vi "Triggered Tasks-Stop.vi"(8 "error in (no error)":errorcluster, 11 "Logging queue element":T1={"Imaging Protocol"=enum."Live Imaging", "Number of Trials"=0, "Frame Size"=512, "# Averaged frames"=0, "Dwell time (us)"=0.0, "Index of Z-plane"=0, "Timelapse?"=FALSE, "Logging process is active"=FALSE, "Speed logging enabled"=FALSE, "tdms file ref"=refnum, "path"=path "", "Trial Number"=0, "Expected # points acquired"=FALSE, "Manually stopped"=FALSE, "Last trial"=FALSE, "Ch0 data"=[], "Ch1 data"=[], "Ref Data"=[], "Ref Frame Time"=[], "Image Time"=[], "Continuous Time"=[], "Ref X Length"=0, "Ref Y Length"=0, "# Ref Averaged frames"=0, "Ref Dwell time (us)"=0.0, "Points acquired"={"Ch0 last trial"=0, "Ch1 last trial"=0, "All trials"=0}, "HW Timings File"=refnum} {"Ref Dwell time (us)" format="%#.6g"; "Frame Size" items=["100X100"=100, "128X128"=128, "200X200"=200, "256X256"=256, "512X512"=512, "1024x1024"=1024, "2048x2048"=2048]; "Dwell time (us)" format="%#.6g"}) -> (0 "error out":errorcluster)   [LabVIEW 2020]
uses:
  Typedefs/Logging queue element.ctl
  Typedefs/Imaging Protocols enum.ctl
  Typedefs/Frame Size.ctl
  Typedefs/Acquired points count.ctl
  Typedefs/Read Write Enum.ctl
  Typedefs/fgv_actions.ctl
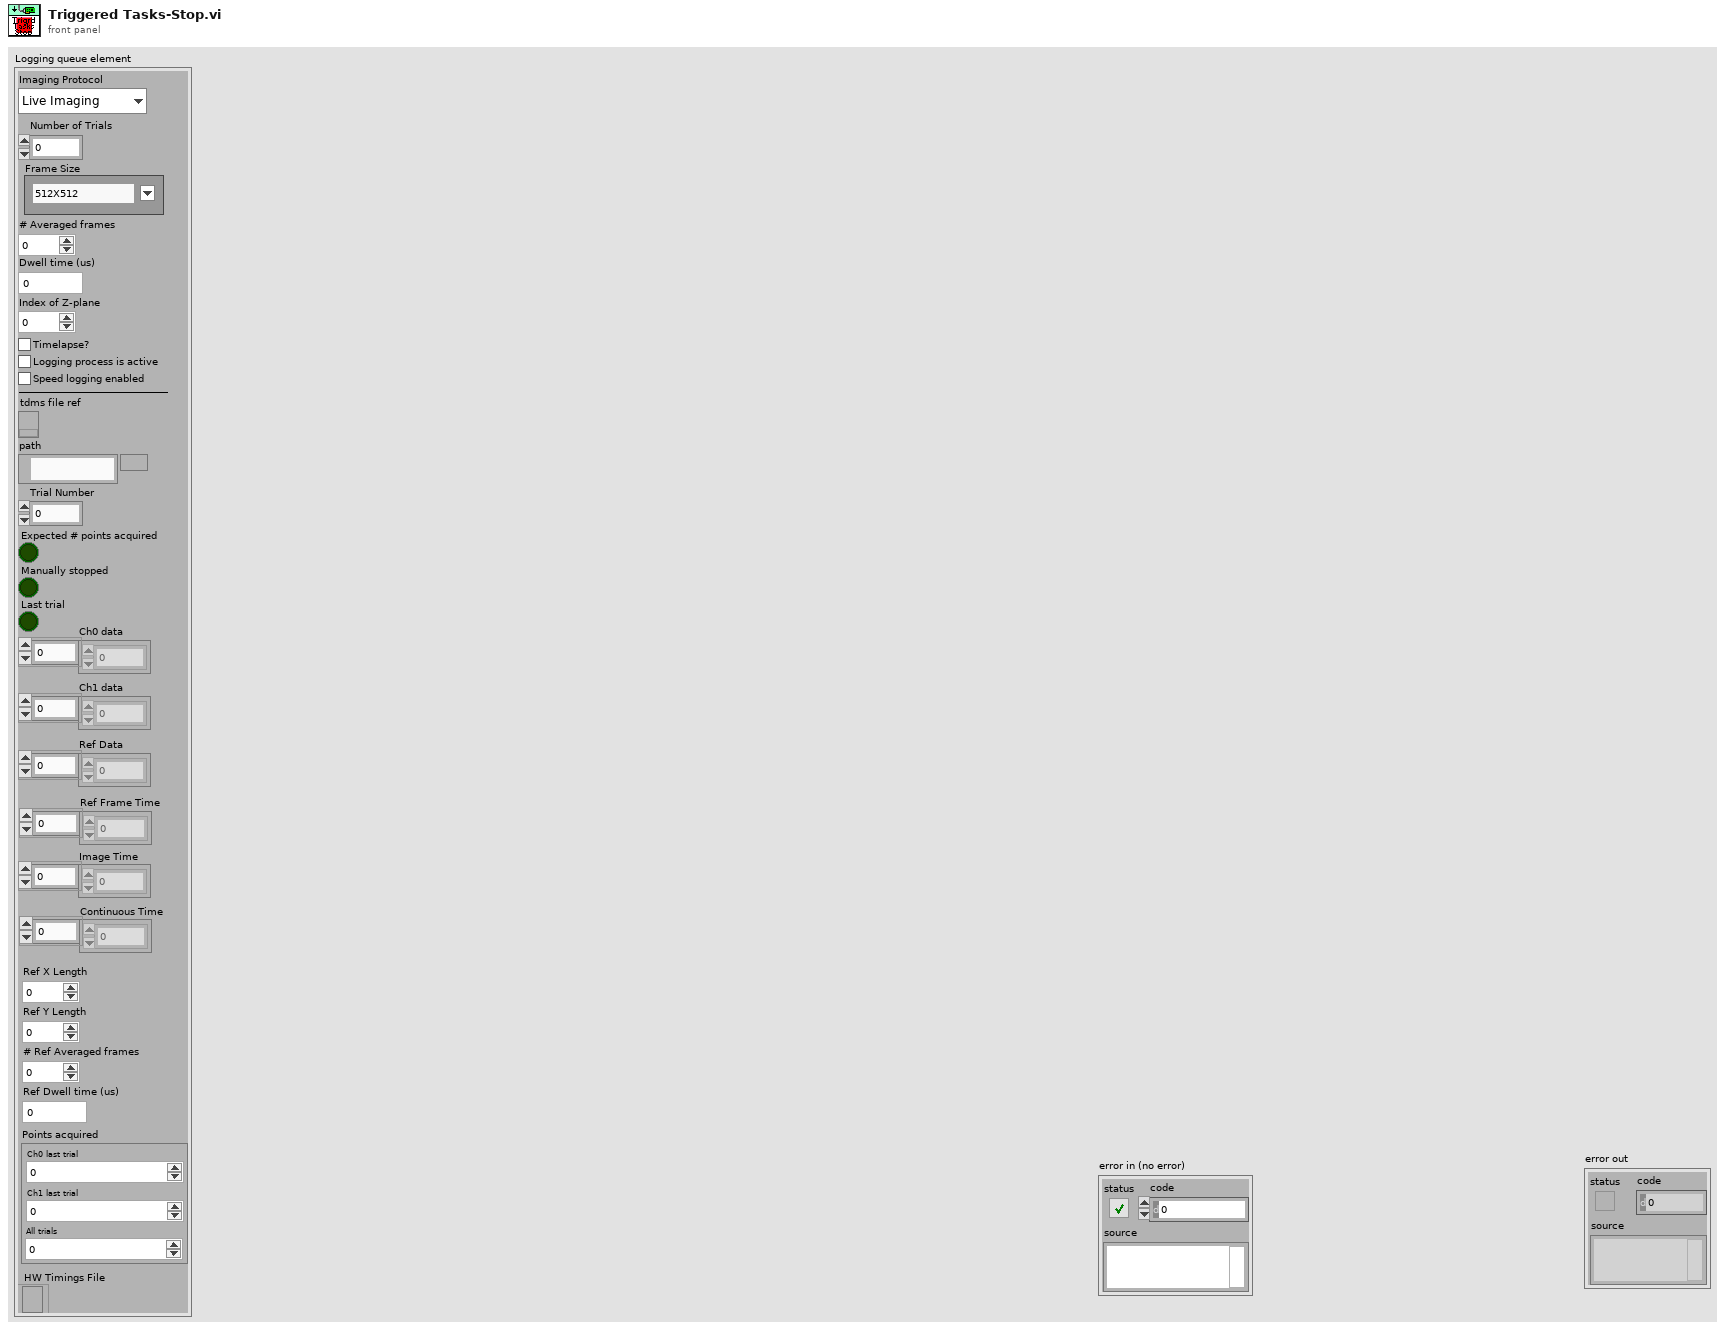
[diagram p1: front panel]
types:
  T1 = typedef "Logging queue element.ctl" = cluster{"Imaging Protocol":T2, "Number of Trials":u16, "Frame Size":T3, "# Averaged frames":u16, "Dwell time (us)":dbl, "Index of Z-plane":i32, "Timelapse?":bool, "Logging process is active":bool, "Speed logging enabled":bool, "tdms file ref":refnum<k34>, "path":path, "Trial Number":i32, "Expected # points acquired":bool, "Manually stopped":bool, "Last trial":bool, "Ch0 data":u32[], "Ch1 data":u32[], "Ref Data":u32[], "Ref Frame Time":u64[], "Image Time":u64[], "Continuous Time":u64[], "Ref X Length":u16, "Ref Y Length":u16, "# Ref Averaged frames":u16, "Ref Dwell time (us)":dbl, "Points acquired":T4, "HW Timings File":refnum<file>}
  T2 = typedef "Imaging Protocols enum.ctl" = enum16{"AOL Z-Stack", "Motor Z Stack", "Parameter Sweep", "Functional Acquisition", "Single Plane Acquisition", "Volume Acquisition", "Live Imaging", "Live Plane Imaging", "Live Volume Imaging"}
  T3 = typedef "Frame Size.ctl" = u16
  T4 = typedef "Acquired points count.ctl" = cluster{"Ch0 last trial":u64, "Ch1 last trial":u64, "All trials":u64}
  T5 = typedef "Read Write Enum.ctl" = enum16{"Read", "Write"}
  T6 = typedef "fgv_actions.ctl" = enum16{"Get", "Set"}
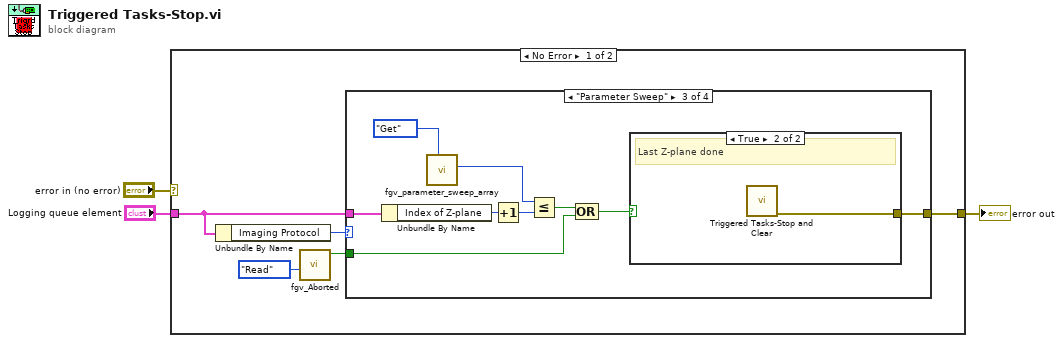
[diagram p0: block diagram]
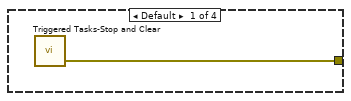
[diagram p2: hidden frame]
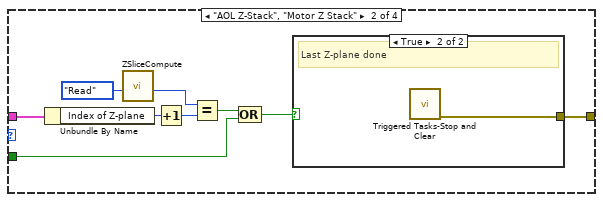
[diagram p3: hidden frame]
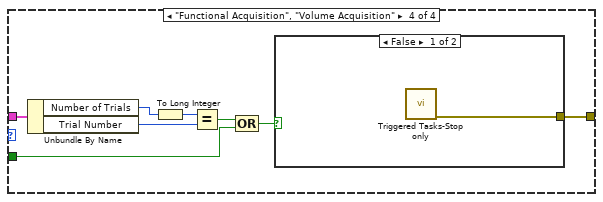
[diagram p6: hidden frame]
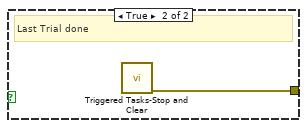
[diagram p7: hidden frame]
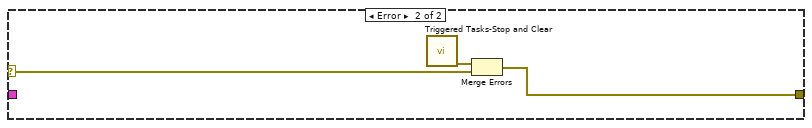
[diagram p8: hidden frame]
diagram:
  n1 = case shown="No Error" "error in (no error)" {
    selector: "error in (no error)" -> [_ w41]
    tunnel: [w8 w40] -> w2
    tunnel: "Logging queue element" -> [w6 _]
    frame No Error {
      n2 = Unbundle By Name(w6) -> ("Imaging Protocol"=w7:T2)
      n3 = call "fgv_Aborted.vi"("Function"=Read_Write_Enum."Read") -> ("Funct Acq Aborted?"=w4:bool)  [unwired: 9 in, 1 out]
      n4 = case shown="\"Parameter Sweep\"" w7 {
        tunnel: w6 -> [_ w18 w28 w37]
        tunnel: [w9 w13 w25 w36] -> w8
        tunnel: w4 -> [_ w10 w22 w30]
        frame Default {
          n5 = call "Triggered Tasks-Stop and Clear.vi"() -> ("error out"=w9:errorcluster)  [unwired: 11 in]
        }
        frame "AOL Z-Stack", "Motor Z Stack" {
          n6 = Unbundle By Name(w18) -> ("Index of Z-plane"=w17:i32)
          n7 = call "ZSliceCompute.vi"("Function"=Read_Write_Enum."Read") -> ("# of Z-planes"=w15:i32)  [unwired: 7 in, 3 out]
          n8 = Increment(x=w17) -> (x+1=w14:i32)
          n9 = Equal?(x=w15, y=w14) -> (x = y?=w12:bool)
          n10 = Compound Arithmetic op=OR(w12, w10) -> (w11:bool)
          n11 = case shown="True" w11 {
            tunnel: [_ w19] -> w13
            frame False {
              # "Not the last plane"
            }
            frame True {
              # "Last Z-plane done"
              n12 = call "Triggered Tasks-Stop and Clear.vi"() -> ("error out"=w19:errorcluster)  [unwired: 11 in]
            }
          }
        }
        frame "Parameter Sweep" {
          n13 = Unbundle By Name(w28) -> ("Index of Z-plane"=w27:i32)
          n14 = call "fgv_parameter_sweep_array.vi"("FGV Actions"=fgv_actions."Get") -> ("Par. Sweep Array Size O/P"=w20:i32)  [unwired: 8 in, 2 out]
          n15 = Increment(x=w27) -> (x+1=w26:i32)
          n16 = Less Or Equal?(x=w20, y=w26) -> (x <= y?=w24:bool)
          n17 = Compound Arithmetic op=OR(w24, w22) -> (w23:bool)
          n18 = case shown="True" w23 {
            tunnel: [_ w29] -> w25
            frame False {
              # "Not the last plane"
            }
            frame True {
              # "Last Z-plane done"
              n19 = call "Triggered Tasks-Stop and Clear.vi"() -> ("error out"=w29:errorcluster)  [unwired: 11 in]
            }
          }
        }
        frame "Functional Acquisition", "Volume Acquisition" {
          n20 = Unbundle By Name(w37) -> ("Number of Trials"=w34:u16, "Trial Number"=w35:i32)
          n21 = To Long Integer(number=w34) -> (32bit integer=w33:i32)
          n22 = Equal?(x=w33, y=w35) -> (x = y?=w32:bool)
          n23 = Compound Arithmetic op=OR(w32, w30) -> (w31:bool)
          n24 = case shown="False" w31 {
            tunnel: [w38 w39] -> w36
            frame False {
              n25 = call "Triggered Tasks-Stop only.vi"() -> ("error out"=w38:errorcluster)  [unwired: 11 in]
            }
            frame True {
              # "Last Trial done"
              n26 = call "Triggered Tasks-Stop and Clear.vi"() -> ("error out"=w39:errorcluster)  [unwired: 11 in]
            }
          }
        }
      }
    }
    frame Error {
      n27 = call "Triggered Tasks-Stop and Clear.vi"() -> ("error out"=w42:errorcluster)  [unwired: 11 in]
      n28 = Merge Errors(w42, w41) -> (w40:errorcluster)
    }
  }
  "error out" <- w2
